vi "SIM Registry Init Header.vi"(4 "Num Cont States":i32=-1, 5 "Discrete Id":i32=-1, 6 "State Idx":i32=-1, 7 "Input Width":i32, 8 "Discrete State Idx":i32=-1, 9 "Num Disc States":i32=-1, 11 "Output Width":i32) -> (3 "Node Header":T1)   [LabVIEW 2017]
uses:
  <vilib>/Simulation/Implementation/Shared/SIM Registry.llb/SIM Registry Node Header.ctl
panel:
  in  "Has ZC?":bool
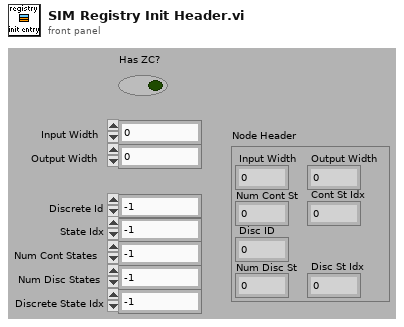
[diagram p1: front panel]
types:
  T1 = typedef "SIM Registry Node Header.ctl" = cluster{"Input Width":i32, "Disc ID":i32, "Num Cont St":i32, "Cont St Idx":i32, "Num Disc St":i32, "Disc St Idx":i32, "Output Width":i32}
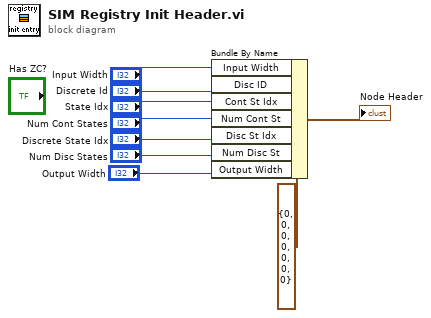
[diagram p0: block diagram]
diagram:
  n1 = Bundle By Name(cluster=T1 {"Input Width"=0, "Disc ID"=0, "Num Cont St"=0, "Cont St Idx"=0, "Num Disc St"=0, "Disc St Idx"=0, "Output Width"=0} ("Node Header"), "Input Width"="Input Width", "Disc ID"="Discrete Id", "Cont St Idx"="State Idx", "Num Cont St"="Num Cont States", "Disc St Idx"="Discrete State Idx", "Num Disc St"="Num Disc States", "Output Width"="Output Width") -> (→"Node Header":T1)
